vi "InitSingleStack.vi"(8 "ActionStack in":refnum<class "ActionStack.lvclass">) -> (1 "Action Stack":refnum<class "ActionStack.lvclass">[](array[class]))   [LabVIEW 2024]
uses:
  ActionStack.lvclass
  ActionStack.lvclass/ActionStack.ctl
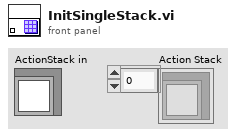
[diagram p1: front panel]
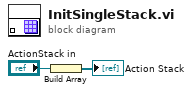
[diagram p0: block diagram]
diagram:
  n1 = Build Array("ActionStack in") -> (→"Action Stack":refnum<class "ActionStack.lvclass">[])
